vi "string to profibus channel.vi"(10 "channel data":string, 11 "identifier":string) -> (3 "Profibus channel":refnum<class "Profibus channel.lvclass">)   [LabVIEW 2013, in "Profibus channel.lvclass"]
uses:
  Profibus channel.lvclass
  <vilib>/NI/Tag Bus/tag/Data Type.ctl
  <vilib>/NI/Tag Bus Module Framework/channel/channel classification.ctl
  <vilib>/NI/Tag Bus/tag/tag descriptor.lvclass/tag descriptor.ctl
  <vilib>/NI/Tag Bus Module Framework/channel/TBM channel.lvclass/TBM channel.ctl
  Profibus channel.lvclass/Profibus channel.ctl
  <vilib>/NI/Tag Bus Module Framework/root configuration/TBM configuration.lvclass
  <vilib>/NI/Tag Bus/tag/tag descriptor.lvclass
  <vilib>/NI/Tag Bus Module Framework/channel/TBM channel.lvclass
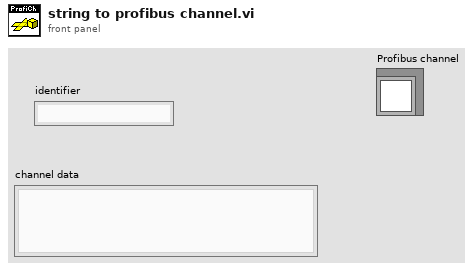
[diagram p1: front panel]
types:
  T1 = typedef "TBM channel.lvclass/channel classification.ctl" = enum16{"input data", "output data", "processing parameter", "processing result"}
  T2 = typedef "tag bus.lvlib/tag descriptor.lvclass/Data Type.ctl" = enum16{"Double", "Single", "I64", "I32", "I16", "I8", "U64", "U32", "U16", "U8", "Boolean", "String", "Array of Double", "Array of Single", "Array of I64", "Array of I32", "Array of I16", "Array of I8", "Array of U64", "Array of U32", "Array of U16", "Array of U8", "Array of Boolean", "Array of String"}
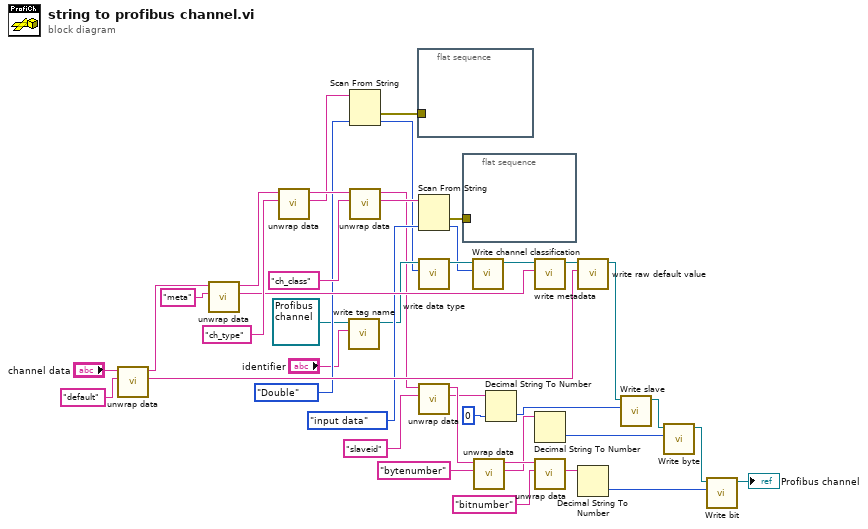
[diagram p0: block diagram]
diagram:
  n1 = call <vilib>:"unwrap data.vi"("identifier"="default", "data to unwrap"="channel data") -> ("unwrapped data"=w32:string, "remaining string"=w41:string)  [unwired: 8 in]
  n2 = call <vilib>:"unwrap data.vi"("identifier"="meta", "data to unwrap"=w41) -> ("unwrapped data"=w33:string, "remaining string"=w37:string)  [unwired: 8 in]
  n3 = call <vilib>:"unwrap data.vi"("identifier"="ch_type", "data to unwrap"=w37) -> ("unwrapped data"=w31:string, "remaining string"=w38:string)  [unwired: 8 in]
  n4 = call <vilib>:"write tag name.vi"("name"="identifier", "system tag in"=refnum<class "Profibus channel.lvclass"> refnum ("Profibus channel.lvclass")) -> ("system tag out"=w23:refnum<class "Profibus channel.lvclass">)  [unwired: 8 in, 1 out]
  n5 = Scan From String(input string=w31, default 1=Data_Type."Double" ("data type")) -> (error out=w27:errorcluster, output 1=w22:T2)  [unwired: 3 in, 2 out]
  n6 = call <vilib>:"unwrap data.vi"("identifier"="ch_class", "data to unwrap"=w38) -> ("unwrapped data"=w29:string, "remaining string"=w11:string)  [unwired: 8 in]
  n7 = flat-sequence {
    tunnel: w27 -> [_]
    frame #0 {
    }
  }
  n8 = Scan From String(input string=w29, default 1=channel_classification."input data" ("channel classification")) -> (error out=w26:errorcluster, output 1=w20:T1)  [unwired: 3 in, 2 out]
  n9 = call <vilib>:"write data type.vi"("data type"=w22, "system tag in"=w23) -> ("system tag out"=w21:refnum<class "Profibus channel.lvclass">)  [unwired: 8 in, 1 out]
  n10 = call <vilib>:"unwrap data.vi"("identifier"="slaveid", "data to unwrap"=w11) -> ("unwrapped data"=w3:string, "remaining string"=w12:string)  [unwired: 8 in]
  n11 = flat-sequence {
    tunnel: w26 -> [_]
    frame #0 {
    }
  }
  n12 = call <vilib>:"Write channel classification.vi"("channel classification"=w20, "channel in"=w21) -> ("channel out"=w19:refnum<class "Profibus channel.lvclass">)  [unwired: 8 in, 1 out]
  n13 = call <vilib>:"unwrap data.vi"("identifier"="bytenumber", "data to unwrap"=w12) -> ("unwrapped data"=w4:string, "remaining string"=w13:string)  [unwired: 8 in]
  n14 = Decimal String To Number(string=w3, default (0L)=i8 0 ("default (0 I32)")) -> (number=w2:i8)  [unwired: 1 in, 1 out]
  n15 = call <vilib>:"write metadata.vi"("metadata"=w33, "system tag in"=w19) -> ("system tag out"=w34:refnum<class "Profibus channel.lvclass">)  [unwired: 8 in, 1 out]
  n16 = Decimal String To Number(string=w4) -> (number=w5:i32)  [unwired: 2 in, 1 out]
  n17 = call <vilib>:"unwrap data.vi"("identifier"="bitnumber", "data to unwrap"=w13) -> ("unwrapped data"=w7:string)  [unwired: 8 in, 1 out]
  n18 = call <vilib>:"write raw default value.vi"("raw default"=w32, "system tag in"=w34) -> ("system tag out"=w15:refnum<class "Profibus channel.lvclass">)  [unwired: 8 in, 1 out]
  n19 = Decimal String To Number(string=w7) -> (number=w6:i32)  [unwired: 2 in, 1 out]
  n20 = call "Write slave.vi"("slave"=w2, "Profibus channel in"=w15) -> ("Profibus channel out"=w16:refnum<class "Profibus channel.lvclass">)  [unwired: 8 in, 1 out]
  n21 = call "Write byte.vi"("byte"=w5, "Profibus channel in"=w16) -> ("Profibus channel out"=w17:refnum<class "Profibus channel.lvclass">)  [unwired: 8 in, 1 out]
  n22 = call "Write bit.vi"("bit"=w6, "Profibus channel in"=w17) -> ("Profibus channel out"=→"Profibus channel":refnum<class "Profibus channel.lvclass">)  [unwired: 8 in, 1 out]
